vi "Actor Core.vi"(8 "error in":errorcluster, 11 "Measure Pulse in":refnum<class "Measure Pulse.lvclass">) -> (0 "error out":errorcluster, 3 "Actor out":refnum<class "Actor.lvclass">)   [LabVIEW 2015, in "Measure Pulse.lvclass"]
doc: "(<B>Filename</B>: Actor Framework.lvlib:Actor.lvclass:Actor Core.vi)\n\nReceives messages to the actor, reacts to them, and initiates any error handling that may shut the actor down.\n\nDescendant classes may override this VI to append parallel tasks for the actor to complete while it handles messages. Overrides use the Call Parent Method node."
uses:
  Measure Pulse.lvclass
  <vilib>/ActorFramework/Actor/Actor.lvclass
  Queued Listbox/Queued Listbox.xctl
  Common Measurements/Common Measurements.lvclass
panel:
  in  "Refresh Button":bool
  out "File Path":path
  in  "Write cfg":bool
  in  "Read cfg":bool
  in  "Graph":bool
  out "Running 2":bool=TRUE
  out "Running":bool=TRUE
  in  "Disarm":bool
  in  "Arm":bool
  in  "Stop":bool
  in  "Run":bool
  in  "Parameters":cluster{"Pulse duration":dbl}={"Pulse duration"=-1.0} {"Pulse duration" format="%#_6p"}
  in  "Monitor":string[](xcontrol)
  in  "Proccess":string[](xcontrol)
  in  "Acquire Pulse":string[](xcontrol)
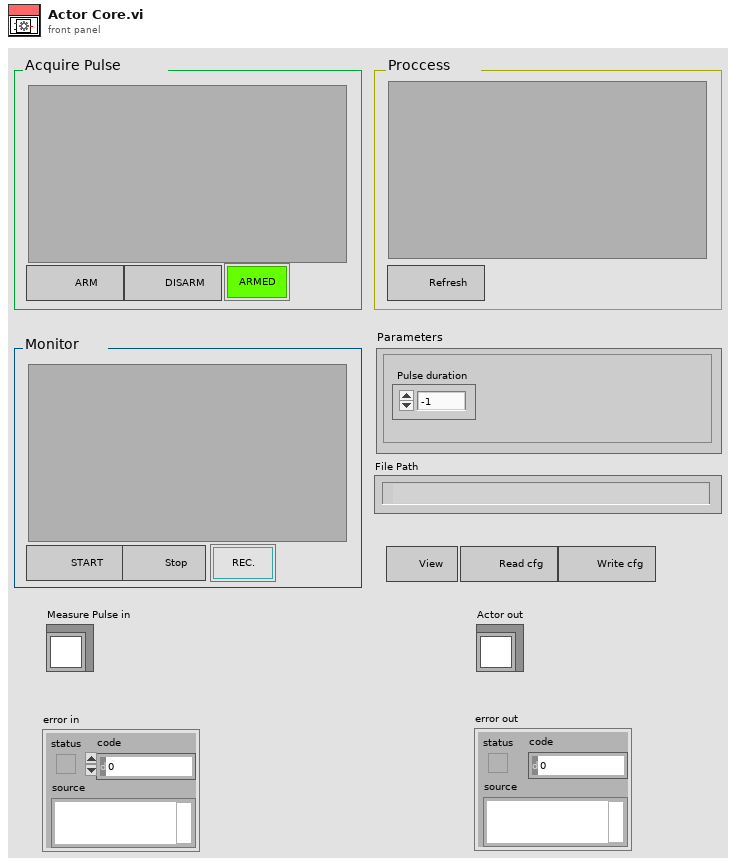
[diagram p1: front panel]
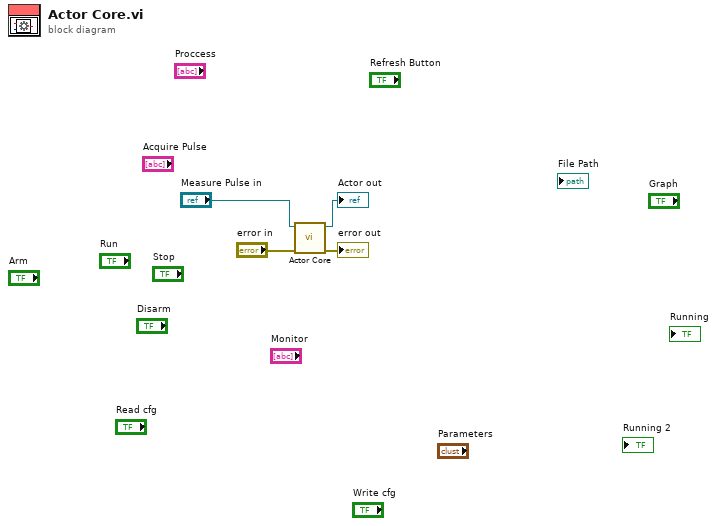
[diagram p0: block diagram]
diagram:
  n1 = call-parent "Actor Core.vi"("error in"="error in", "Mag Lab Measure Base in"="Measure Pulse in") -> ("error out"=→"error out":errorcluster, "Actor out"=→"Actor out":refnum<class "Actor.lvclass">)  [unwired: 8 in]
